vi "rethinkdb_query_run.vi"(4 "global options (key,val)":string[][](array[string]), 6 "timeout ms (10000)":i32=10000, 8 "error in (no error)":errorcluster, 9 "query_type (START)":T1, 10 "reql_id in":u32 format="%08x", 11 "rethinkdb in":refnum<k5>) -> (0 "error out":errorcluster, 2 "reql_id out":u32 format="%08x", 3 "rethinkdb out":refnum<k5>)   [LabVIEW 2017]
uses:
  ql2proto/ql2proto_query_type.ctl
  ast/ast_reql_cache.vi
  <vilib>/Utility/error.llb/Error Cluster From Error Code.vi
  ql2proto/ql2proto_query_type_encode.vi
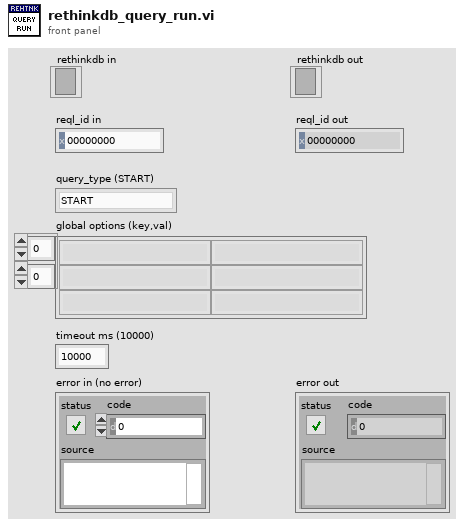
[diagram p1: front panel]
types:
  T1 = typedef "ql2proto_query_type.ctl" = enum8{"START", "CONTINUE", "STOP", "NOREPLY_WAIT", "SERVER_INFO", "invalid"}
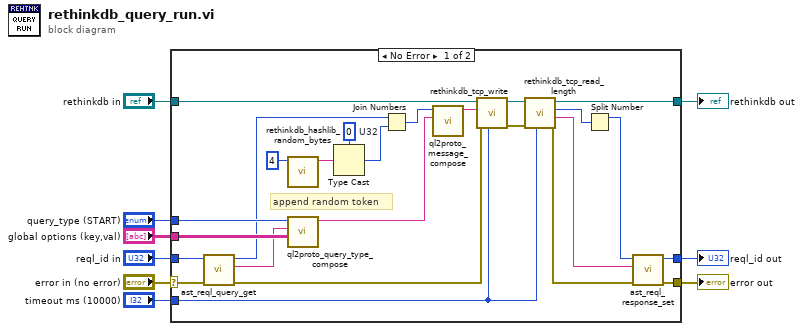
[diagram p0: block diagram]
diagram:
  n1 = case shown="No Error" "error in (no error)" {
    selector: "error in (no error)" -> [w31 w37]
    tunnel: "reql_id in" -> [w11 w35]
    tunnel: "rethinkdb in" -> [w34 w36]
    tunnel: [w19 w36] -> w6
    tunnel: "timeout ms (10000)" -> [w20 _]
    tunnel: [w14 w37] -> w4
    tunnel: "query_type (START)" -> [w33 _]
    tunnel: "global options (key,val)" -> [w23 _]
    tunnel: [w10 w35] -> w1
    frame No Error {
      w27 = u32 0  # U32
      # "append random token"
      n2 = call "ast_reql_query_get.vi"("error in (no error)"=w31, "reql_id in"=w11) -> ("error out"=w30:errorcluster, "query"=w17:string, "reql_id out"=w16:u32)  [unwired: 7 in]
      n3 = call "rethinkdb_hashlib_random_bytes.vi"("length (18bytes)"=4) -> ("random bytes"=w28:string)  [unwired: 10 in]
      n4 = call "ql2proto_query_type_compose.vi"("global options (key,val)"=w23, "query"=w17, "query_type"=w33) -> ("tcp_write"=w25:string)  [unwired: 8 in]
      n5 = Type Cast(type=w27, x=w28) -> (*(type *) &x=w26:u32)
      n6 = Join Numbers(hi=w16, lo=w26) -> ((hi.lo)=w24:u64)
      n7 = call "ql2proto_message_compose.vi"("query"=w25, "token"=w24) -> ("tcp_write"=w32:string)  [unwired: 9 in]
      n8 = call "rethinkdb_tcp_write.vi"("timeout ms (10000)"=w20, "error in (no error)"=w30, "tcp_write"=w32, "rethinkdb in"=w34) -> ("error out"=w21:errorcluster, "rethinkdb out"=w22:refnum<k5>)  [unwired: 5 in, 1 out]
      n9 = call "rethinkdb_tcp_read_length.vi"("timeout ms (10000)"=w20, "error in (no error)"=w21, "rethinkdb in"=w22) -> ("error out"=w15:errorcluster, "response"=w12:string, "token"=w18:u64, "rethinkdb out"=w19:refnum<k5>)  [unwired: 5 in]
      n10 = Split Number(x=w18) -> (hi(x)=w13:u32)  [unwired: 1 out]
      n11 = call "ast_reql_response_set.vi"("error in (no error)"=w15, "response"=w12, "reql_id in"=w13) -> ("error out"=w14:errorcluster, "reql_id out"=w10:u32)  [unwired: 7 in]
    }
    frame Error {
    }
  }
  "error out" <- w4
  "rethinkdb out" <- w6
  "reql_id out" <- w1
